vi "JSON-ClusterForInstructionsDB.vi"(6 "Table":string, 8 "error in (no error)":errorcluster, 11 "Payload":string) -> (0 "error out":errorcluster, 3 "Cluster Out":T1(array[cluster]))   [LabVIEW 2014]
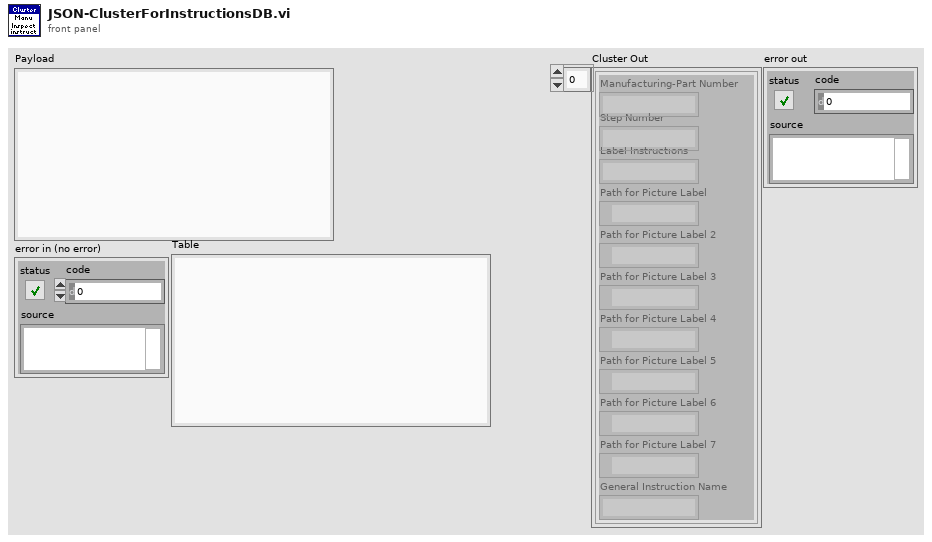
[diagram p1: front panel]
types:
  T1 = cluster{"Manufacturing-Part Number":string, "Step Number":string, "Label Instructions":string, "Path for Picture Label":path, "Path for Picture Label 2":path, "Path for Picture Label 3":path, "Path for Picture Label 4":path, "Path for Picture Label 5":path, "Path for Picture Label 6":path, "Path for Picture Label 7":path, "General Instruction Name":string}[]
  T2 = cluster{"Manufacturing-Part Number":string, "Array of Cluster Data":cluster{"Label Instructions":string, "Path for Picture Label":path, "Path for Picture Label 2":path, "Path for Picture Label 3":path, "Path for Picture Label 4":path, "Path for Picture Label 5":path, "Path for Picture Label 6":path, "Path for Picture Label 7":path, "Label Instructions 2":string, "Label Instructions 3":string}[], "Type of Insert":i32}
  T3 = cluster{"General Process Name":string, dbl, "Manufacturing-Label":cluster{"Label Instructions":string, "Path for Picture Label":path, "Path for Picture Label 2":path, "Path for Picture Label 3":path, "Path for Picture Label 4":path, "Path for Picture Label 5":path, "Path for Picture Label 6":path, "Path for Picture Label 7":path}}
  T4 = cluster{"Label Instructions":string, "Path for Picture Label":path, "Path for Picture Label 2":path, "Path for Picture Label 3":path, "Path for Picture Label 4":path, "Path for Picture Label 5":path, "Path for Picture Label 6":path, "Path for Picture Label 7":path, "Label Instructions 2":string, "Label Instructions 3":string}[]
  T5 = cluster{"Manufacturing-Part Number":string, "Label Instructions 2":string, "Label Instructions":string, "Path for Picture Label":path, "Path for Picture Label 2":path, "Path for Picture Label 3":path, "Path for Picture Label 4":path, "Path for Picture Label 5":path, "Path for Picture Label 6":path, "Path for Picture Label 7":path, "Label Instructions 3":string}
  T6 = cluster{"Label Instructions":string, "Path for Picture Label":path, "Path for Picture Label 2":path, "Path for Picture Label 3":path, "Path for Picture Label 4":path, "Path for Picture Label 5":path, "Path for Picture Label 6":path, "Path for Picture Label 7":path}
  T7 = cluster{"General Process Name":string, string, "Label Instructions":string, "Path for Picture Label":path, "Path for Picture Label 2":path, "Path for Picture Label 3":path, "Path for Picture Label 4":path, "Path for Picture Label 5":path, "Path for Picture Label 6":path, "Path for Picture Label 7":path, "y":string}
  T8 = cluster{"General Process Name":string, string, "Label Instructions":string, "Path for Picture Label":path, "Path for Picture Label 2":path, "Path for Picture Label 3":path, "Path for Picture Label 4":path, "Path for Picture Label 5":path, "Path for Picture Label 6":path, "Path for Picture Label 7":path, "y":string}[]
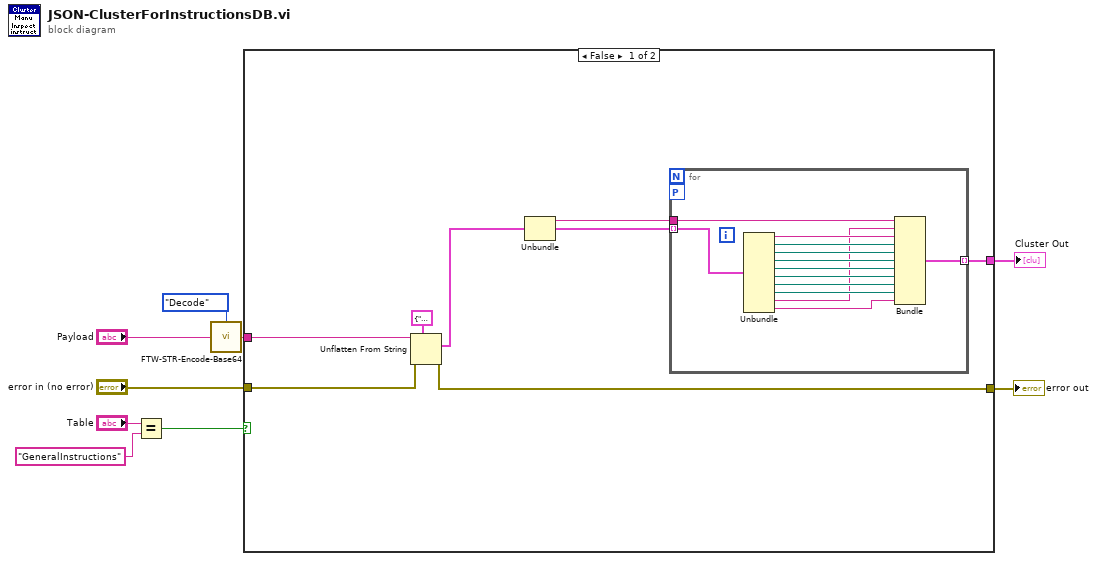
[diagram p0: block diagram]
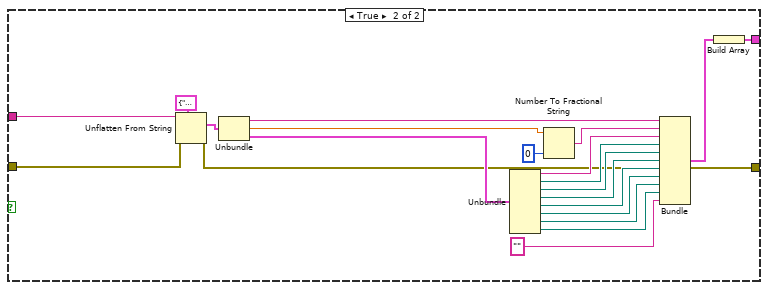
[diagram p2: hidden frame]
diagram:
  n1 = Equal?(x="Table", y="GeneralInstructions") -> (x = y?=w2:bool)
  n2 = call "FTW-STR-Encode-Base64.vi"("Input"="Payload", "Direction"=enum16{"Encode", "Decode"}."Decode") -> ("Output"=w8:string)
  n3 = case shown="False" w2 {
    tunnel: w8 -> [w17 w37]
    tunnel: "error in (no error)" -> [w13 w36]
    tunnel: [w12 w34] -> w5
    tunnel: [w10 w33] -> w1
    frame False {
      n4 = Unflatten From String(type=T2 {"Manufacturing-Part Number"="", "Array of Cluster Data"=[], "Type of Insert"=0} ("cluster"), binary string=w17, error in (no error)=w13) -> (value=w16:T2, error out=w10:errorcluster)  [unwired: 2 in, 1 out]
      n5 = Unbundle(w16) -> ("Manufacturing-Part Number"=w14:string, "Array of Cluster Data"=w15:T4)  [unwired: 1 out]
      n6 = for {
        tunnel: w15 -> [w30] mode=indexing
        tunnel: w14 -> [w29]
        workers-P: _ -> [_]
        tunnel: [w20] -> w12 mode=indexing
        n7 = Unbundle(w30) -> ("Label Instructions"=w28:string, "Path for Picture Label"=w27:path, "Path for Picture Label 2"=w26:path, "Path for Picture Label 3"=w25:path, "Path for Picture Label 4"=w24:path, "Path for Picture Label 5"=w23:path, "Path for Picture Label 6"=w22:path, "Path for Picture Label 7"=w21:path, "Label Instructions 2"=w19:string, "Label Instructions 3"=w18:string)
        n8 = Bundle("Manufacturing-Part Number"=w29, "Label Instructions 2"=w19, "Label Instructions"=w28, "Path for Picture Label"=w27, "Path for Picture Label 2"=w26, "Path for Picture Label 3"=w25, "Path for Picture Label 4"=w24, "Path for Picture Label 5"=w23, "Path for Picture Label 6"=w22, "Path for Picture Label 7"=w21, "Label Instructions 3"=w18) -> (w20:T5)  [unwired: 1 in]
      }
    }
    frame True {
      n9 = Unflatten From String(type=T3 {"General Process Name"="", 0.0, "Manufacturing-Label"={"Label Instructions"="", "Path for Picture Label"=path "", "Path for Picture Label 2"=path "", "Path for Picture Label 3"=path "", "Path for Picture Label 4"=path "", "Path for Picture Label 5"=path "", "Path for Picture Label 6"=path "", "Path for Picture Label 7"=path ""}} ("cluster"), binary string=w37, error in (no error)=w36) -> (value=w39:T3, error out=w33:errorcluster)  [unwired: 2 in, 1 out]
      n10 = Unbundle(w39) -> ("General Process Name"=w38:string, w49:dbl, "Manufacturing-Label"=w50:T6)
      n11 = Unbundle(w50) -> ("Label Instructions"=w41:string, "Path for Picture Label"=w42:path, "Path for Picture Label 2"=w43:path, "Path for Picture Label 3"=w44:path, "Path for Picture Label 4"=w45:path, "Path for Picture Label 5"=w46:path, "Path for Picture Label 6"=w47:path, "Path for Picture Label 7"=w48:path)
      n12 = Number To Fractional String(number=w49, precision (6)=i16 0) -> (F-format string=w40:string)  [unwired: 2 in]
      n13 = Bundle("General Process Name"=w38, w40, "Label Instructions"=w41, "Path for Picture Label"=w42, "Path for Picture Label 2"=w43, "Path for Picture Label 3"=w44, "Path for Picture Label 4"=w45, "Path for Picture Label 5"=w46, "Path for Picture Label 6"=w47, "Path for Picture Label 7"=w48, "y"="") -> (w35:T7)  [unwired: 1 in]
      n14 = Build Array(w35) -> (w34:T8)
    }
  }
  "Cluster Out" <- w5
  "error out" <- w1
